vi "Switch_Static Dig Path Gen Initialize.vi"(0 "Switch Resource Name":refnum<k15>, 5 "Topology Name":T2="2527/2-Wire Dual 16x1 Mux", 11 "error in":errorcluster) -> (4 "Switch Handle Out":refnum<k15>, 6 "Module Characteristics":T1, 15 "error out":errorcluster)   [LabVIEW 2021, in "Switch_Static Digital Path Generation.lvlib"]
doc: "Initializes and resets an NI-SWITCH session based on the module selected in the <B>Switch Resource Name</B> control and the topology to be applied. Returns an output session handle and the maximum switching voltage and current characteristics from the module."
uses:
  Switch_Static Digital Path Generation.lvlib
  <instrlib>/niSwitch/niSwitch.llb/niSwitch Topologies.ctl
  Typedefs/Module Characteristics.ctl
panel:
  # "Inputs"
  # "Outputs"
  # "Overview:\nThis VI interacts with the NI-SWITCH driver to initialize and reset an NI SWITCH module, provides a corresponding Switch Handle Output and the maximum switching module characteristics based on the Topology and Switch Resource Name.\n\nHardware Requirements: A PXI Switch Module\n\nSoftware Requirements: NI-SWITCH 2022 Q4 or above\n\nInstructions:\nSelect your Switch Module resource name in the drop down control and select the Topology you want to apply based on your needs\n\nNote: The \"Switch Handle Out\" indicator will be used by the Configure & Measure and Close API functions"
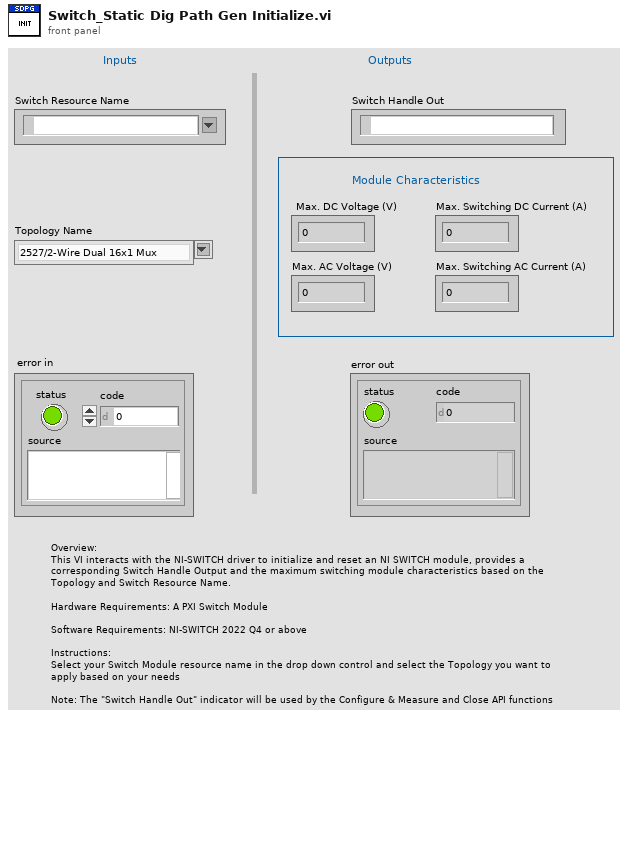
[diagram p1: front panel]
types:
  T1 = typedef "Switch_Static Digital Path Generation.lvlib/Module Characteristics.ctl" = cluster{" Max. DC Voltage (V)":dbl, "Max. Switching DC Current (A)":dbl, "Max. AC Voltage (V)":dbl, "Max. Switching AC Current (A)":dbl}
  T2 = typedef "niSwitch Topologies.ctl" = string
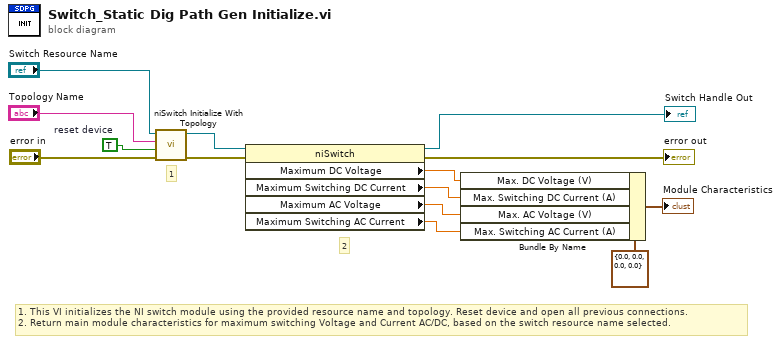
[diagram p0: block diagram]
diagram:
  w7 = TRUE  # reset device
  # "2"
  # "1. This VI initializes the NI switch module using the provided resource name and topology. Reset device and open all previous connections.\n2. Return main module characteristics for maximum switching Voltage and Current AC/DC, based on the switch resource name selected."
  # "1"
  n1 = call <instrlib>:"niSwitch Initialize With Topology.vi"("error in (no error)"="error in", "reset device (boolean value)"=w7, "topology name"="Topology Name", "resource name"="Switch Resource Name") -> ("error out"=w9:errorcluster, "instrument handle out"=w11:refnum<k15>)  [unwired: 1 in, 5 out]
  n2 = property class="niSwitch"(reference=w11, error in=w9) -> (reference out=→"Switch Handle Out":refnum<k15>, error out=→"error out":errorcluster, "Maximum DC Voltage"=w6:dbl, "Maximum Switching DC Current"=w5:dbl, "Maximum AC Voltage"=w4:dbl, "Maximum Switching AC Current"=w3:dbl)
  n3 = Bundle By Name(cluster=T1 {" Max. DC Voltage (V)"=0.0, "Max. Switching DC Current (A)"=0.0, "Max. AC Voltage (V)"=0.0, "Max. Switching AC Current (A)"=0.0} ("Module Characteristics"), "Max. DC Voltage (V)"=w6, "Max. Switching DC Current (A)"=w5, "Max. AC Voltage (V)"=w4, "Max. Switching AC Current (A)"=w3) -> (→"Module Characteristics":T1)
